vi "peak comb -- interpolate - complex plane - V3.vi"(8 "peaks are known -- parameters":T1={"Def Gamma (kHz)"=0.0, "dV"=0.0, "time in Gamma (sec)"=0.0, "phi-star"=0.0, "all peaks (kHz)"=[564.0, 649.0, 987.0, 1133.0, 1214.0, 1585.0, 1763.0, 1823.0, 1880.0, 1899.0, 2032.0, 2138.0, 2221.0, 2270.0, 2350.0, 2456.0, 2580.0, 2634.0, 2831.0, 2960.0, 2965.0, 3131.0, 3328.0, 3469.0, 3553.0, 0.0, 3615.0, 3734.0, 0.0, 0.0, 0.0, 4236.0, 4300.0, 4331.0], "delta t (sec)"=0.0, "default step (Hz)"=0.0, "all gamma (kHz)"=[564.0, 649.0, 987.0, 1133.0, 1214.0, 1585.0, 1763.0, 1823.0, 1880.0, 1899.0, 2032.0, 2138.0, 2221.0, 2270.0, 2350.0, 2456.0, 2580.0, 2634.0, 2831.0, 2960.0, 2965.0, 3131.0, 3328.0, 3469.0, 3553.0, 0.0, 3615.0, 3734.0, 0.0, 0.0, 0.0, 4236.0, 4300.0, 4331.0], "peaks OK"=FALSE, "gamma OK"=FALSE, "near omega (kHz)"=0.0, "near gamma (kHz)"=0.0, "min step (Hz)"=10000.0, "max step(Hz)"=0.01, "min gamma (kHz)"=0.01, "all time in gamma (sec)"=[], "time in gamma OK"=FALSE}, 11 "freq (kHz)":dbl) -> (0 "peaks are known -- parameters out":T1={"Def Gamma (kHz)"=1.0, "dV"=0.0, "time in Gamma (sec)"=10.0, "phi-star"=3.14, "all peaks (kHz)"=[564.0, 649.0, 987.0, 1133.0, 1214.0, 1585.0, 1763.0, 1823.0, 1880.0, 1899.0, 2032.0, 2138.0, 2221.0, 2270.0, 2350.0, 2456.0, 2580.0, 2634.0, 2831.0, 2960.0, 2965.0, 3131.0, 3328.0, 3469.0, 3553.0, 0.0, 3615.0, 3734.0, 0.0, 0.0, 0.0, 4236.0, 4300.0, 4331.0], "delta t (sec)"=0.0, "default step (Hz)"=1.0, "all gamma (kHz)"=[564.0, 649.0, 987.0, 1133.0, 1214.0, 1585.0, 1763.0, 1823.0, 1880.0, 1899.0, 2032.0, 2138.0, 2221.0, 2270.0, 2350.0, 2456.0, 2580.0, 2634.0, 2831.0, 2960.0, 2965.0, 3131.0, 3328.0, 3469.0, 3553.0, 0.0, 3615.0, 3734.0, 0.0, 0.0, 0.0, 4236.0, 4300.0, 4331.0], "peaks OK"=FALSE, "gamma OK"=FALSE, "near omega (kHz)"=0.0, "near gamma (kHz)"=0.0, "min step (Hz)"=10000.0, "max step(Hz)"=0.01, "min gamma (kHz)"=0.01, "all time in gamma (sec)"=[], "time in gamma OK"=FALSE}, 1 "near omega (kHz)":dbl, 2 "near gamma (kHz)":dbl, 3 "delta-F (Hz)":dbl=-1.0)   [LabVIEW 2012]
uses:
  next chunk -- parameters.ctl
  Q - not nan -- real.vi
panel:
  in  "max step(Hz)":dbl=10000.0
  in  "min step (Hz)":dbl=0.01
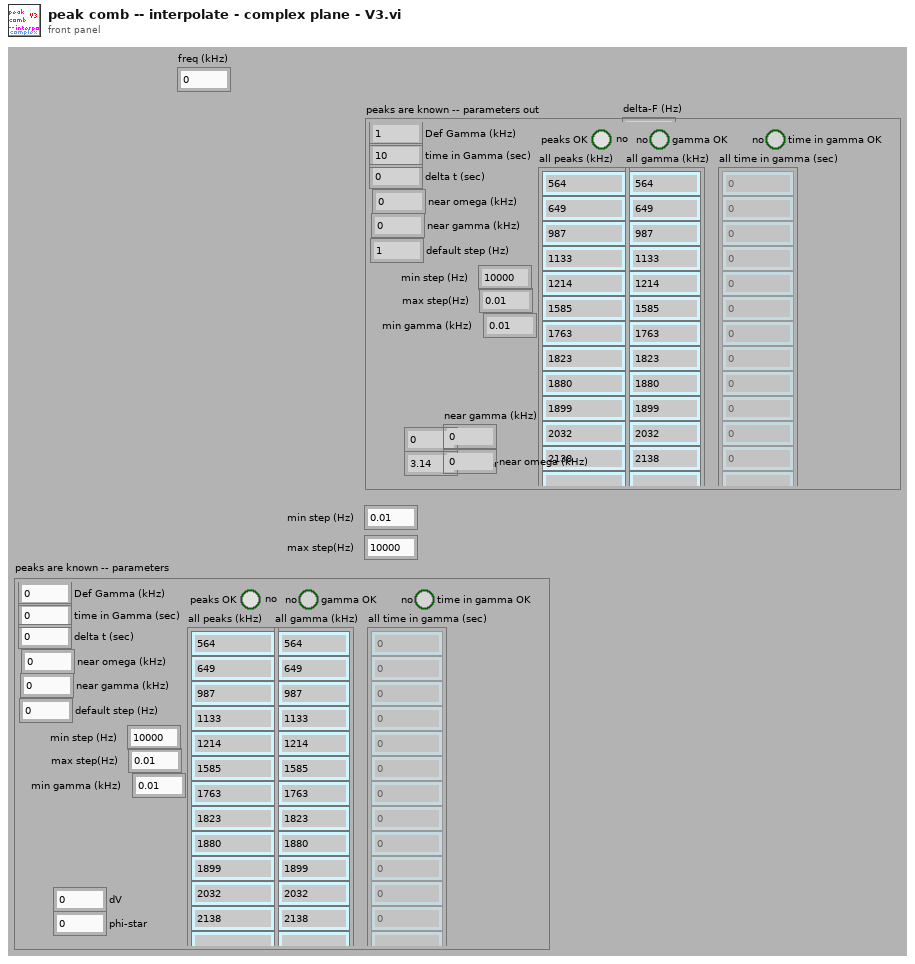
[diagram p1: front panel]
types:
  T1 = typedef "next chunk -- parameters.ctl" = cluster{"Def Gamma (kHz)":dbl, "dV":dbl, "time in Gamma (sec)":dbl, "phi-star":dbl, "all peaks (kHz)":dbl[], "delta t (sec)":dbl, "default step (Hz)":dbl, "all gamma (kHz)":dbl[], "peaks OK":bool, "gamma OK":bool, "near omega (kHz)":dbl, "near gamma (kHz)":dbl, "min step (Hz)":dbl, "max step(Hz)":dbl, "min gamma (kHz)":dbl, "all time in gamma (sec)":dbl[], "time in gamma OK":bool}
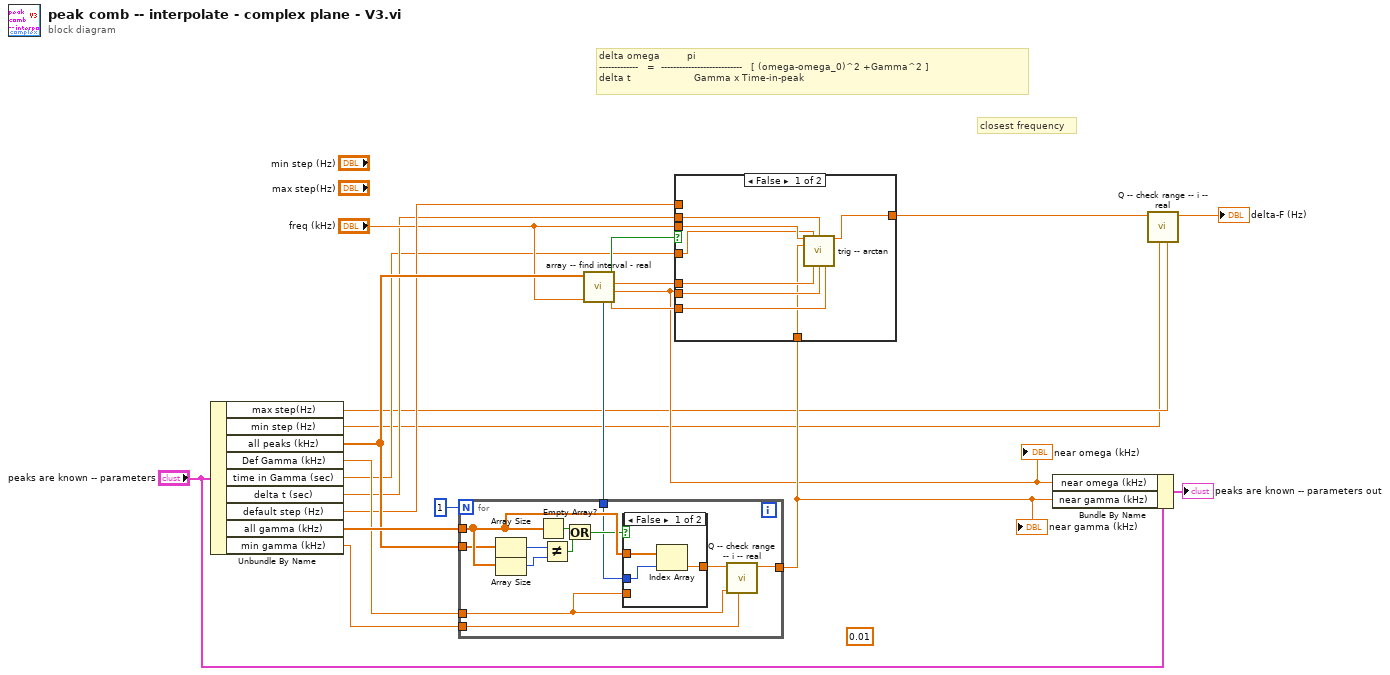
[diagram p0: block diagram]
diagram:
  (unwired) 0.01 ("lower")
  # "closest frequency"
  # "delta omega         pi\n-------------   =  ---------------------------   [ (omega-omega_0)^2 +Gamma^2 ] \ndelta t                     Gamma x Time-in-peak"
  n1 = Unbundle By Name("peaks are known -- parameters") -> ("max step(Hz)"=w4:dbl, "min step (Hz)"=w3:dbl, "all peaks (kHz)"=w18:dbl[], "Def Gamma (kHz)"=w20:dbl, "time in Gamma (sec)"=w10:dbl, "delta t (sec)"=w11:dbl, "default step (Hz)"=w16:dbl, "all gamma (kHz)"=w21:dbl[], "min gamma (kHz)"=w2:dbl)
  n2 = call "array -- find interval - real.vi"("number"="freq (kHz)", "array"=w18) -> ("omega plus (kHz)"=w14:dbl, "omega zero (kHz)"=w6:dbl, "omega minus (kHz)"=w15:dbl, "out of range?"=w17:bool, "closest element index"=w13:i32)  [unwired: 4 in, 1 out]
  "near omega (kHz)" <- w6
  n3 = for {
    N: 1 -> [_]
    tunnel: w21 -> [w32]
    tunnel: w20 -> [w26]
    tunnel: w18 -> [w25]
    tunnel: w13 -> [w24]
    tunnel: [w23] -> w7
    tunnel: w2 -> [w22]
    n4 = Array Size(array=w25) -> (size(s)=w30:i32)
    n5 = Array Size(array=w32) -> (size(s)=w31:i32)
    n6 = Empty Array?(array=w32) -> (empty?=w29:bool)
    n7 = Not Equal?(x=w30, y=w31) -> (x != y?=w28:bool)
    n8 = Or(x=w29, y=w28) -> (x .or. y?=w27:bool)
    n9 = case shown="False" w27 {
      tunnel: w24 -> [w36 _]
      tunnel: [w35 w37] -> w33
      tunnel: w32 -> [w34 _]
      tunnel: w26 -> [_ w37]
      frame False {
        n10 = Index Array(array=w34, index=w36) -> (element=w35:dbl)
      }
      frame True {
      }
    }
    n11 = call "Q -- check range -- i -- real.vi"("lower"=w22, "default"=w26, "number"=w33) -> ("number in range"=w23:dbl)  [unwired: 6 in, 2 out]
  }
  "near gamma (kHz)" <- w7
  n12 = case shown="False" w17 {
    tunnel: [w38 w46] -> w9
    tunnel: w16 -> [_ w46]
    tunnel: w15 -> [w45 _]
    tunnel: w6 -> [w44 _]
    tunnel: w14 -> [w43 _]
    tunnel: w7 -> [w42 _]
    tunnel: "freq (kHz)" -> [w41 _]
    tunnel: w11 -> [w40 _]
    tunnel: w10 -> [w39 _]
    frame False {
      n13 = call "trig -- arctan.vi"("omega (kHz)"=w41, "time in Gamma (sec)"=w39, "delta t (sec)"=w40, "gamma (kHz)"=w42, "omega minus (kHz)"=w45, "omega zero (kHz)"=w44, "omega plus (kHz)"=w43) -> ("freq step (Hz)"=w38:dbl)  [unwired: 8 in]
    }
    frame True {
    }
  }
  n14 = Bundle By Name(cluster="peaks are known -- parameters", "near omega (kHz)"=w6, "near gamma (kHz)"=w7) -> (→"peaks are known -- parameters out":T1)
  n15 = call "Q -- check range -- i -- real.vi"("upper"=w4, "lower"=w3, "number"=w9) -> ("number in range"=→"delta-F (Hz)":dbl)  [unwired: 6 in, 2 out]
